vi "_JKISMQFGV.vi"(6 "Operation":T3, 8 "Error in":errorcluster caption="Error in (no error)", 9 "create if not found? (T)":bool=TRUE, 11 "Name(\"\" to use uuid) in":string) -> (0 "Error out":errorcluster, 1 "Boolean":bool, 2 "Name":string[](array[string]), 3 "Array":T1[](array[typedef]))   [LabVIEW 2014, in "JKI State Machine++.lvlib"]
uses:
  JKI State Machine++.lvlib
  _JKISMQFGVOPER.ctl
  _JKISMQ.ctl
  Typedef/_Cross JKISM State Data.ctl
  Typedef/_JKISM_MSG_TYPE.ctl
  Typedef/_Cross JKISM State Response.ctl
  Typedef/_JKISM_MODE.ctl
  Typedef/_JKISM Status Change Event Data.ctl
  FGV-BroadcastRegistry/Operation-BroadcastRegistry.ctl
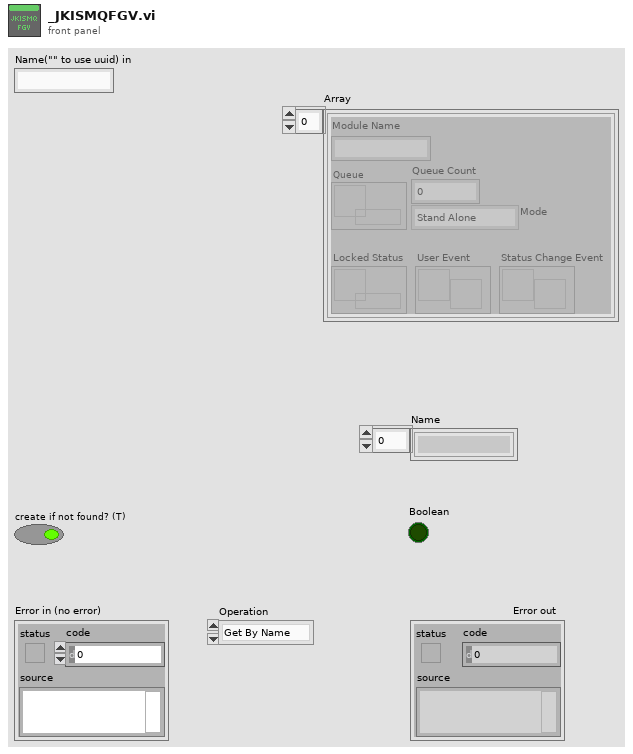
[diagram p1: front panel]
types:
  T1 = typedef "JKI State Machine++.lvlib/_JKISMQ.ctl" = cluster{"Module Name":string, "Queue":refnum<queue>, "Locked Status":refnum<data-value>, "Mode":T2, "User Event":refnum<user-event>, "Queue Count":i32, "Status Change Event":refnum<user-event>}
  T2 = typedef "JKI State Machine++.lvlib/_JKISM_MODE.ctl" = enum16{"Stand Alone", "JKISM", "Action Worker"}
  T3 = typedef "JKI State Machine++.lvlib/_JKISMQFGVOPER.ctl" = enum16{"Get By Name", "List", "Check If Name Exists", "Release", "Module Status", "Create Status Event Handler", "Destroy Status Event Handler"}
  T4 = typedef "JKI State Machine++.lvlib/Operation-BroadcastRegistry.ctl" = enum16{"Delete Source Module", "Delete Target Module", "Remove Module", "Register", "Unregister", "Check"}
  T5 = typedef "JKI State Machine++.lvlib/_JKISM Status Change Event Data.ctl" = cluster{"ModuleName":string, "Status":string, "Arguments":string}
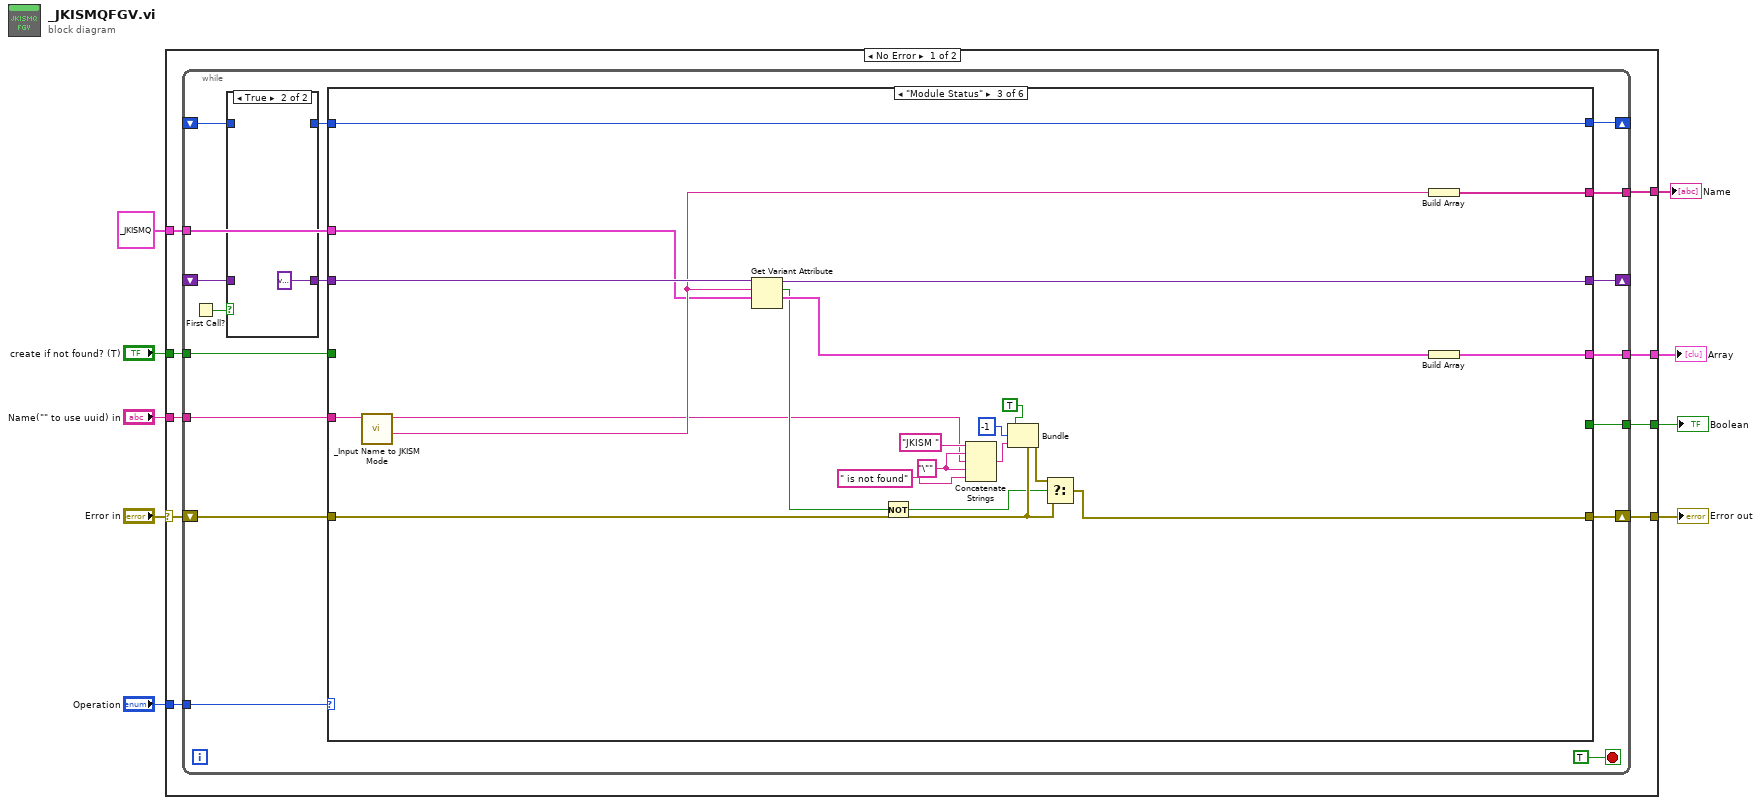
[diagram p0: block diagram]
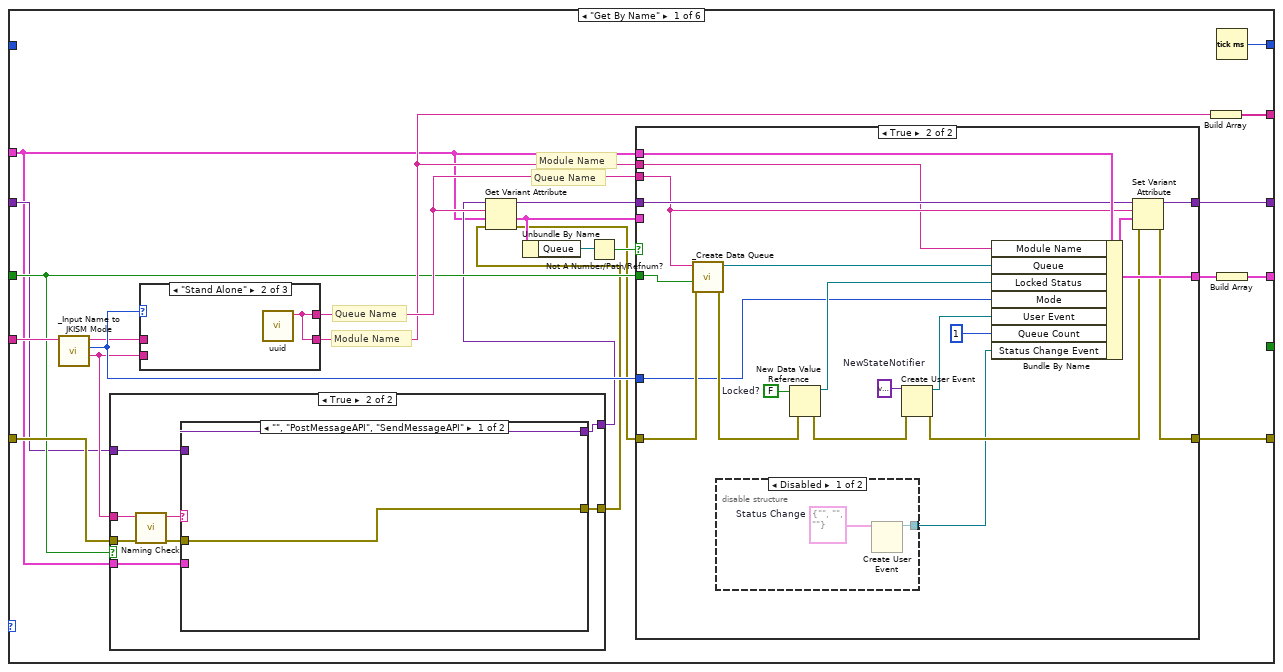
[diagram p3: hidden frame]
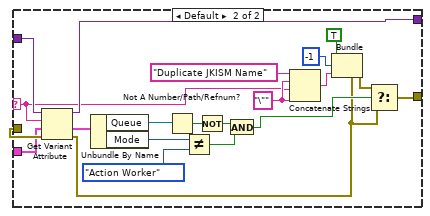
[diagram p5: hidden frame]
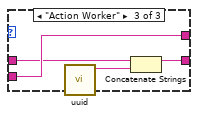
[diagram p7: hidden frame]
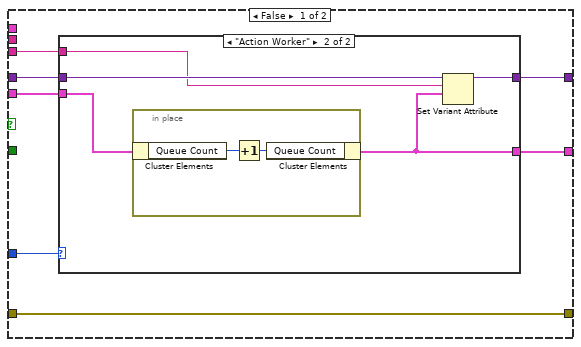
[diagram p8: hidden frame]
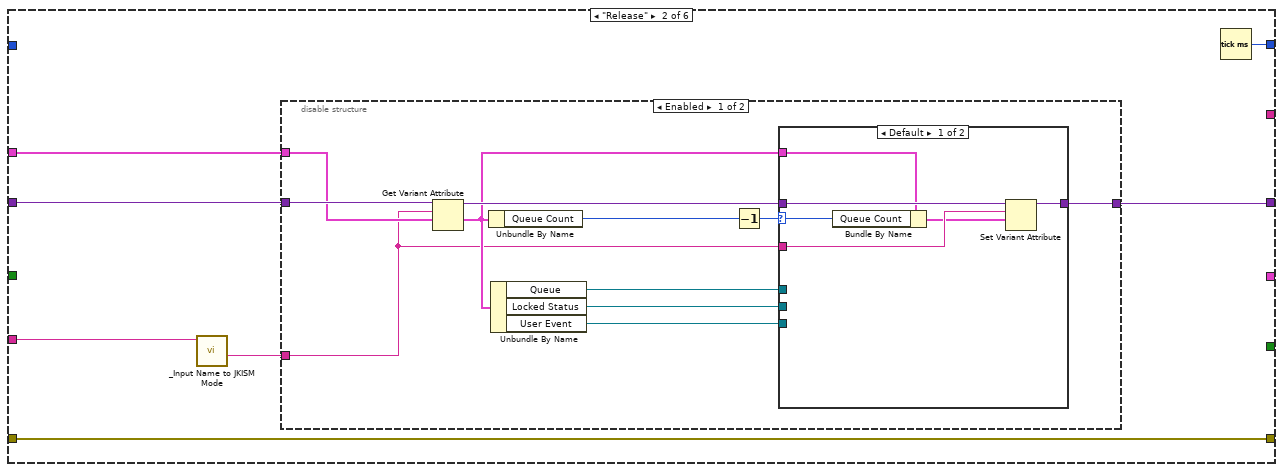
[diagram p11: hidden frame]
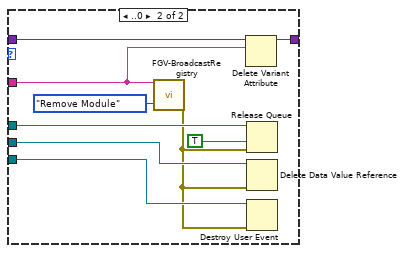
[diagram p12: hidden frame]
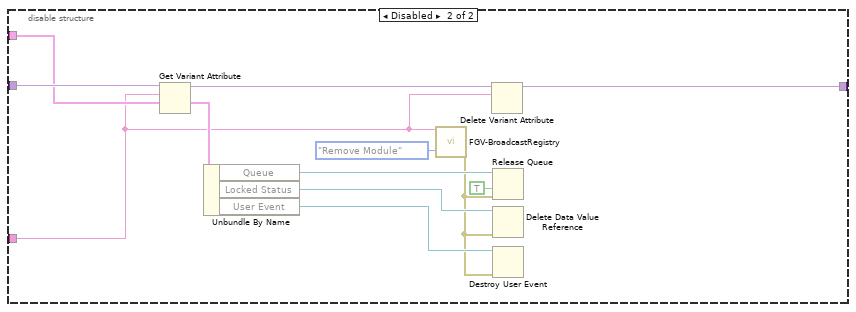
[diagram p13: hidden frame]
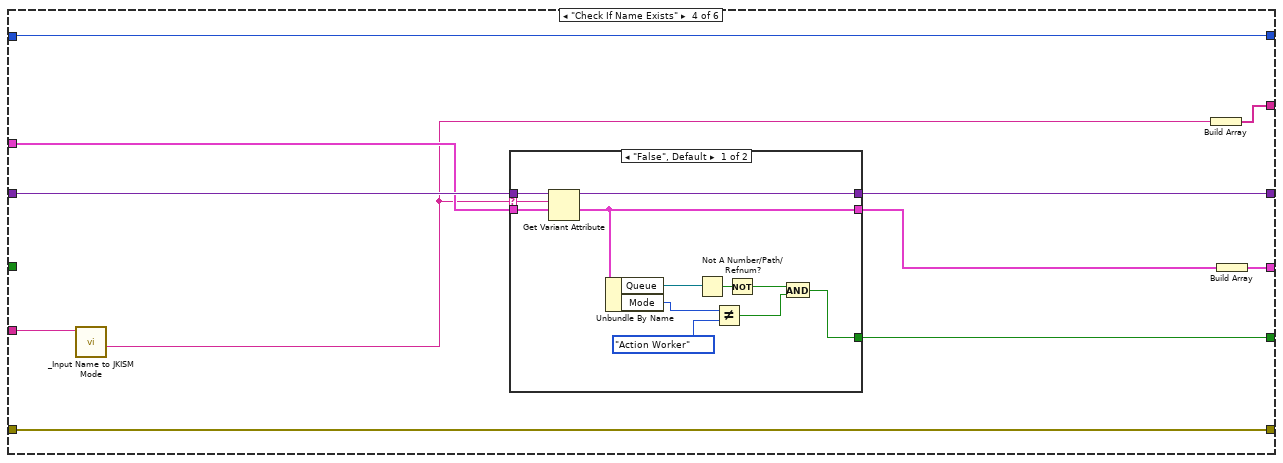
[diagram p14: hidden frame]
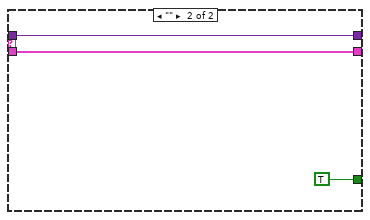
[diagram p15: hidden frame]
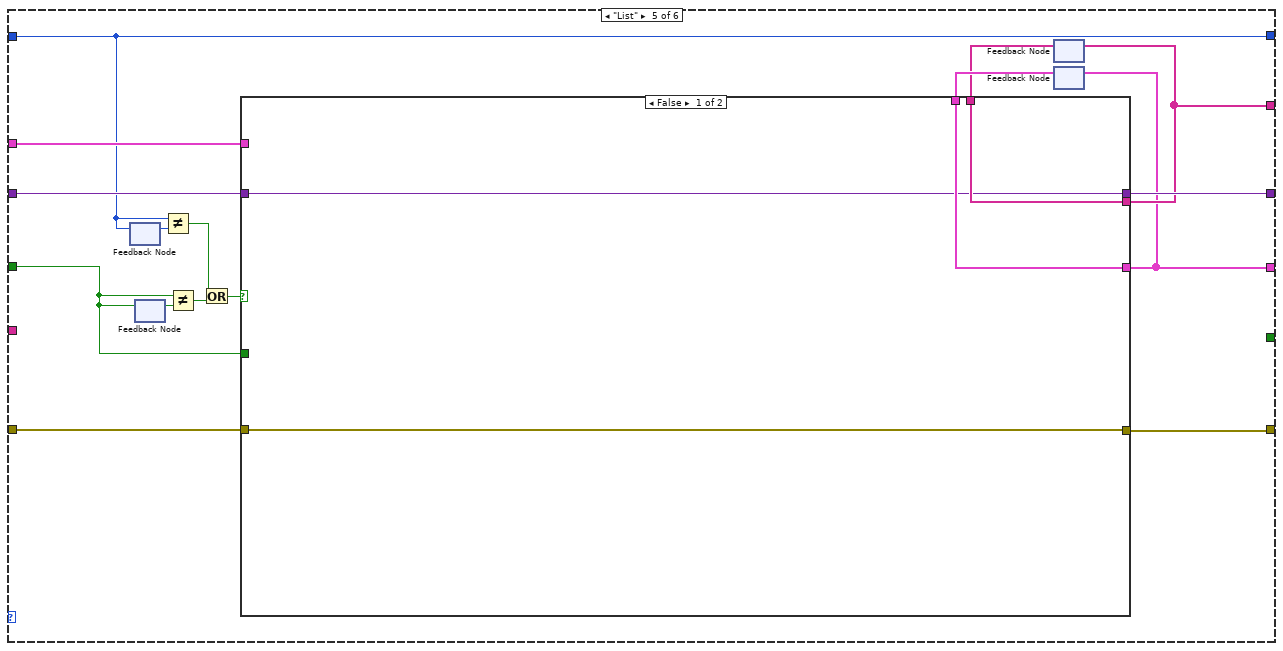
[diagram p16: hidden frame]
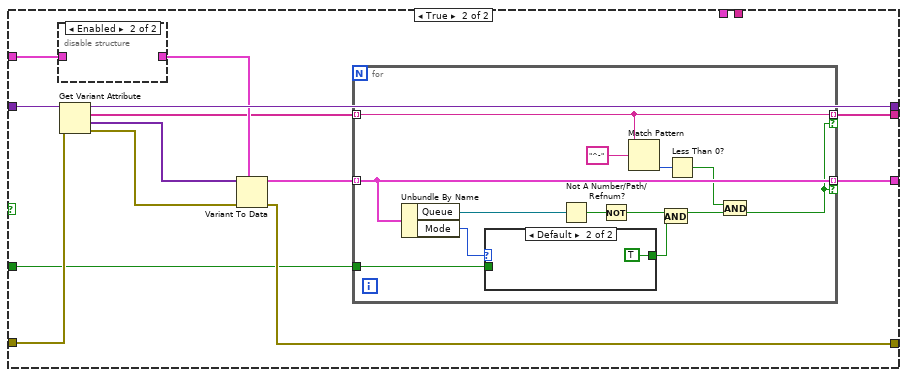
[diagram p17: hidden frame]
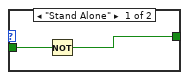
[diagram p18: hidden frame]
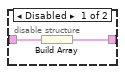
[diagram p19: hidden frame]
diagram:
  n1 = case shown="No Error" "Error in" {
    selector: "Error in" -> [w15 w285]
    tunnel: "Operation" -> [w18 _]
    tunnel: "Name(\"\" to use uuid) in" -> [w17 _]
    tunnel: "create if not found? (T)" -> [w16 _]
    tunnel: [w14 w285] -> w5
    tunnel: [w13 _] -> w4
    tunnel: T1 {"Module Name"="", "Queue"=refnum, "Locked Status"=refnum, "Mode"=enum."Stand Alone", "User Event"=refnum, "Queue Count"=0, "Status Change Event"=refnum} ("JKISMQ") -> [w12 _]
    tunnel: [w11 _] -> w2
    tunnel: [w10 _] -> w1
    frame No Error {
      n2 = while {
        tunnel: w18 -> [w34]
        tunnel: w17 -> [w33]
        tunnel: w16 -> [w32]
        tunnel: [w31] -> w11
        shift-right: [w27] -> _
        shift-left: _ -> [w29]
        shift-right: [w25] -> w14
        shift-left: w15 -> [w26]
        tunnel: [w24] -> w13
        tunnel: w12 -> [w23]
        tunnel: [w22] -> w10
        shift-right: [w21] -> _
        shift-left: _ -> [w19]
        stop <- TRUE stop-if-true
        n3 = First Call?() -> (First Call?: T/F=w30:bool)
        n4 = case shown="True" w30 {
          tunnel: [w37 variant] -> w28
          tunnel: w29 -> [w37 _]
          tunnel: [w36 _] -> w20
          tunnel: w19 -> [w36 _]
          frame False {
          }
          frame True {
          }
        }
        n5 = case shown="\"Module Status\"" w34 {
          tunnel: w33 -> [w52 w141 w203 w207 _ _]
          tunnel: w32 -> [w44 _ _ _ w238 _]
          tunnel: [w54 _ w200 w210 w233 _] -> w31
          tunnel: w28 -> [w43 w144 w204 w215 w246 w284]
          tunnel: [w59 w143 w202 w214 w245 w284] -> w27
          tunnel: w26 -> [w46 w145 w191 w212 w243 w283]
          tunnel: [w55 w145 w188 w212 w242 w283] -> w25
          tunnel: [w53 _ w198 w209 w234 _] -> w24
          tunnel: w23 -> [w41 w142 w196 w211 w244 _]
          tunnel: [_ _ _ w208 _ _] -> w22
          tunnel: w20 -> [_ _ w197 w205 w240 w282]
          tunnel: [w47 w139 w197 w205 w240 w282] -> w21
          frame "Get By Name" {
            # "Module Name"
            # "Queue Name"
            # "Module Name"
            # "Queue Name"
            n6 = call "_Input Name to JKISM Mode.vi"("String"=w52) -> ("Queue Name"=w45:string, "JKISM Mode"=w51:T2, "String(dup)"=w50:string)  [unwired: 8 in]
            n7 = case shown="True" w44 {
              tunnel: w45 -> [_ w65]
              tunnel: [w63 w71] -> w40
              tunnel: w46 -> [w63 w67]
              tunnel: w43 -> [w62 w70]
              tunnel: [w62 w69] -> w42
              tunnel: w41 -> [_ w68]
              frame False {
              }
              frame True {
                n8 = call "Naming Check.vi"("error in (no error)"=w67, "Name(\"\" to use uuid)"=w65) -> ("error out"=w66:errorcluster, "Name(dup)"=w64:string)  [unwired: 8 in]
                n9 = case shown="\"\", \"PostMessageAPI\", \"SendMessageAPI\"" w64 {
                  selector: w64 -> [_ w74]
                  tunnel: [w72 w94] -> w71
                  tunnel: w66 -> [w72 w77]
                  tunnel: w70 -> [w73 w79]
                  tunnel: [w73 w78] -> w69
                  tunnel: w68 -> [_ w75]
                  frame "", "PostMessageAPI", "SendMessageAPI" {
                  }
                  frame Default {
                    w88 = "\"" ("string")
                    n10 = Get Variant Attribute(Variant=w79, name=w74, default value (empty Variant)=w75, error in=w77) -> (duplicate Variant=w78:variant, value=w81:T1, error out=w76:errorcluster)  [unwired: 1 out]
                    n11 = Unbundle By Name(w81) -> ("Queue"=w82:refnum<queue>, "Mode"=w85:T2)
                    n12 = Not A Number/Path/Refnum?(number/path/refnum=w82) -> (NaN/Path/Refnum?=w83:bool)
                    n13 = Not Equal?(x=w85, y=_JKISM_MODE."Action Worker") -> (x != y?=w87:bool)
                    n14 = Not(x=w83) -> (.not. x?=w84:bool)
                    n15 = And(x=w84, y=w87) -> (x .and. y?=w80:bool)
                    n16 = Concatenate Strings("Duplicate JKISM Name" ("String to Prepend to source (\"\")"), w88, w74, w88) -> (w89:string)
                    n17 = Bundle(cluster=w76, "status"=TRUE, "code"=-1, "source"=w89) -> (w93:errorcluster)
                    n18 = Select(t=w93, s=w80, f=w76) -> (s? t:f=w94:errorcluster)
                  }
                }
              }
            }
            n19 = case shown="\"Stand Alone\"" w51 {
              tunnel: [w95 w96 w100] -> w49
              tunnel: [w95 w96 w97] -> w48
              tunnel: w50 -> [w95 _ w99]
              tunnel: w45 -> [_ _ w100]
              frame "JKISM" {
              }
              frame "Stand Alone" {
                n20 = call "uuid.vi"() -> ("UUID"=w96:string)  [unwired: 11 in]
              }
              frame "Action Worker" {
                n21 = call "uuid.vi"() -> ("UUID"=w98:string)  [unwired: 11 in]
                n22 = Concatenate Strings(w99, w98) -> (w97:string)
              }
            }
            n23 = Get Variant Attribute(Variant=w42, name=w49, default value (empty Variant)=w41, error in=w40) -> (duplicate Variant=w60:variant, value=w58:T1, error out=w39:errorcluster)  [unwired: 1 out]
            n24 = Unbundle By Name(w58) -> ("Queue"=w57:refnum<queue>)
            n25 = Not A Number/Path/Refnum?(number/path/refnum=w57) -> (NaN/Path/Refnum?=w56:bool)
            n26 = case shown="True" w56 {
              tunnel: w44 -> [_ w135]
              tunnel: [w103 w129] -> w61
              tunnel: w49 -> [w101 w119]
              tunnel: w41 -> [_ w132]
              tunnel: w60 -> [w104 w131]
              tunnel: [w105 w130] -> w59
              tunnel: w58 -> [w102 _]
              tunnel: w39 -> [w107 w128]
              tunnel: [w107 w126] -> w55
              tunnel: w51 -> [w106 w121]
              tunnel: w48 -> [_ w118]
              frame False {
                n27 = case shown="\"Action Worker\"" w106 {
                  tunnel: [w109 w113] -> w105
                  tunnel: w104 -> [w109 w114]
                  tunnel: [w108 w110] -> w103
                  tunnel: w102 -> [w108 w111]
                  tunnel: w101 -> [_ w112]
                  frame Default {
                  }
                  frame "Action Worker" {
                    n28 = in-place {
                      n29 = in-place-cluster #1(w111) -> ("Queue Count"=w116:i32)
                      n30 = Increment(x=w116) -> (x+1=w115:i32)
                      n31 = in-place-cluster #1("Queue Count"=w115) -> (w110:T1)
                    }
                    n32 = Set Variant Attribute(Variant=w114, name=w112, value=w110) -> (Variant out=w113:variant)  [unwired: 1 in, 2 out]
                  }
                }
              }
              frame True {
                w125 = variant  # NewStateNotifier
                w136 = FALSE  # Locked?
                n33 = call "_Create Data Queue.vi"("error in (no error)"=w128, "create if not found? (T)"=w135, "Name"=w119) -> ("error out"=w127:errorcluster, "Queue out"=w134:refnum<queue>)  [unwired: 6 in, 1 out]
                n34 = disable-structure shown="Disabled" {
                  disable-tunnel: [w137 _] -> w117
                  frame Disabled {
                    w138 = T5 {"ModuleName"="", "Status"="", "Arguments"=""}  # Status Change
                    n35 = Create User Event(user event datatype=w138) -> (user event=w137:refnum<user-event>)  [unwired: 1 in, 1 out]
                  }
                  frame Enabled {
                  }
                }
                n36 = New Data Value Reference(data value=w136, error in=w127) -> (data value reference=w133:refnum<data-value>, error out=w124:errorcluster)
                n37 = Create User Event(user event datatype=w125, error in=w124) -> (user event=w123:refnum<user-event>, error out=w122:errorcluster)
                n38 = Bundle By Name(cluster=w132, "Module Name"=w118, "Queue"=w134, "Locked Status"=w133, "Mode"=w121, "User Event"=w123, "Queue Count"=1, "Status Change Event"=w117) -> (w129:T1)
                n39 = Set Variant Attribute(Variant=w131, name=w119, value=w129, error in=w122) -> (Variant out=w130:variant, error out=w126:errorcluster)  [unwired: 1 out]
              }
            }
            n40 = Build Array(w48) -> (w53:string[])
            n41 = Tick Count (ms)() -> (millisecond timer value=w47:u32)
            n42 = Build Array(w61) -> (w54:T1[])
          }
          frame "Release" {
            n43 = call "_Input Name to JKISM Mode.vi"("String"=w141) -> ("Queue Name"=w140:string)  [unwired: 8 in, 2 out]
            n44 = disable-structure shown="Enabled" {
              disable-tunnel: w144 -> [w153 w180]
              disable-tunnel: [w149 w178] -> w143
              disable-tunnel: w142 -> [w148 w177]
              disable-tunnel: w140 -> [w146 w175]
              frame Enabled {
                n45 = Get Variant Attribute(Variant=w153, name=w146, default value (empty Variant)=w148) -> (duplicate Variant=w150:variant, value=w147:T1)  [unwired: 1 in, 2 out]
                n46 = Unbundle By Name(w147) -> ("Queue Count"=w152:i32)
                n47 = Unbundle By Name(w147) -> ("Queue"=w156:refnum<queue>, "Locked Status"=w155:refnum<data-value>, "User Event"=w154:refnum<user-event>)
                n48 = Decrement(x=w152) -> (x-1=w151:i32)
                n49 = case shown="Default" w151 {
                  selector: w151 -> [w157 _]
                  tunnel: w156 -> [_ w171]
                  tunnel: w155 -> [_ w169]
                  tunnel: w154 -> [_ w168]
                  tunnel: w146 -> [w159 w163]
                  tunnel: w150 -> [w162 w165]
                  tunnel: [w161 w164] -> w149
                  tunnel: w147 -> [w160 _]
                  frame Default {
                    n50 = Bundle By Name(cluster=w160, "Queue Count"=w157) -> (w158:T1)
                    n51 = Set Variant Attribute(Variant=w162, name=w159, value=w158) -> (Variant out=w161:variant)  [unwired: 1 in, 2 out]
                  }
                  frame ..0 {
                    n52 = call "FGV-BroadcastRegistry.vi"("Source"=w163, "Operation"=Operation-BroadcastRegistry."Remove Module") -> ("Error out"=w166:errorcluster)  [unwired: 11 in, 2 out]
                    n53 = Delete Variant Attribute(6:w163, 7:w165) -> (3:w164:variant)  [unwired: 1 in, 2 out]
                    n54 = Release Queue(queue=w171, force destroy? (F)=TRUE, error in (no error)=w166) -> ()  [unwired: 3 out]
                    n55 = Delete Data Value Reference(data value reference=w169, error in=w166) -> ()  [unwired: 2 out]
                    n56 = Destroy User Event(user event=w168, error in=w166) -> ()  [unwired: 1 out]
                  }
                }
              }
              frame Disabled {
                n57 = Get Variant Attribute(Variant=w180, name=w175, default value (empty Variant)=w177) -> (duplicate Variant=w179:variant, value=w176:T1)  [unwired: 1 in, 2 out]
                n58 = Unbundle By Name(w176) -> ("Queue"=w183:refnum<queue>, "Locked Status"=w182:refnum<data-value>, "User Event"=w181:refnum<user-event>)
                n59 = call "FGV-BroadcastRegistry.vi"("Source"=w175, "Operation"=Operation-BroadcastRegistry."Remove Module") -> ("Error out"=w172:errorcluster)  [unwired: 11 in, 2 out]
                n60 = Delete Variant Attribute(6:w175, 7:w179) -> (3:w178:variant)  [unwired: 1 in, 2 out]
                n61 = Release Queue(queue=w183, force destroy? (F)=TRUE, error in (no error)=w172) -> ()  [unwired: 3 out]
                n62 = Delete Data Value Reference(data value reference=w182, error in=w172) -> ()  [unwired: 2 out]
                n63 = Destroy User Event(user event=w181, error in=w172) -> ()  [unwired: 1 out]
              }
            }
            n64 = Tick Count (ms)() -> (millisecond timer value=w139:u32)
          }
          frame "Module Status" {
            w192 = "\"" ("string")
            n65 = call "_Input Name to JKISM Mode.vi"("String"=w203) -> ("Queue Name"=w199:string, "String(dup)"=w186:string)  [unwired: 8 in, 1 out]
            n66 = Get Variant Attribute(Variant=w204, name=w199, default value (empty Variant)=w196) -> (duplicate Variant=w202:variant, found=w190:bool, value=w201:T1)  [unwired: 1 in, 1 out]
            n67 = Not(x=w190) -> (.not. x?=w189:bool)
            n68 = Concatenate Strings("JKISM " ("String to Prepend to source (\"\")"), w192, w186, w192, " is not found" ("string")) -> (w193:string)
            n69 = Bundle(cluster=w191, "status"=TRUE, "code"=-1, "source"=w193) -> (w195:errorcluster)
            n70 = Select(t=w195, s=w189, f=w191) -> (s? t:f=w188:errorcluster)
            n71 = Build Array(w199) -> (w198:string[])
            n72 = Build Array(w201) -> (w200:T1[])
          }
          frame "Check If Name Exists" {
            n73 = call "_Input Name to JKISM Mode.vi"("String"=w207) -> ("Queue Name"=w206:string)  [unwired: 8 in, 2 out]
            n74 = case shown="\"False\", Default" w206 {
              selector: w206 -> [w224 _]
              tunnel: w215 -> [w227 w230]
              tunnel: [w226 w230] -> w214
              tunnel: [w223 w228] -> w213
              tunnel: w211 -> [w225 w228]
              tunnel: [w219 TRUE] -> w208
              frame "False", Default {
                n75 = Get Variant Attribute(Variant=w227, name=w224, default value (empty Variant)=w225) -> (duplicate Variant=w226:variant, value=w223:T1)  [unwired: 1 in, 2 out]
                n76 = Unbundle By Name(w223) -> ("Queue"=w222:refnum<queue>, "Mode"=w218:T2)
                n77 = Not A Number/Path/Refnum?(number/path/refnum=w222) -> (NaN/Path/Refnum?=w221:bool)
                n78 = Not Equal?(x=w218, y=_JKISM_MODE."Action Worker") -> (x != y?=w216:bool)
                n79 = Not(x=w221) -> (.not. x?=w220:bool)
                n80 = And(x=w220, y=w216) -> (x .and. y?=w219:bool)
              }
              frame "" {
              }
            }
            n81 = Build Array(w206) -> (w209:string[])
            n82 = Build Array(w213) -> (w210:T1[])
          }
          frame "List" {
            n83 = feedback-in #2(w240) -> ()
            n84 = feedback #2() -> (w241:u32)  [unwired: 1 in]
            n85 = feedback #3() -> (w239:bool)  [unwired: 1 in]
            n86 = feedback-in #3(w238) -> ()
            n87 = Not Equal?(x=w240, y=w241) -> (x != y?=w236:bool)
            n88 = Not Equal?(x=w238, y=w239) -> (x != y?=w237:bool)
            n89 = Or(x=w236, y=w237) -> (x .or. y?=w235:bool)
            n90 = feedback #4() -> (w231:string[])  [unwired: 1 in]
            n91 = feedback #5() -> (w232:T1[])  [unwired: 1 in]
            n92 = case shown="False" w235 {
              tunnel: w246 -> [w248 w263]
              tunnel: [w248 w262] -> w245
              tunnel: w244 -> [_ w260]
              tunnel: [w249 w256] -> w234
              tunnel: [w250 w255] -> w233
              tunnel: w243 -> [w247 w253]
              tunnel: [w247 w252] -> w242
              tunnel: w238 -> [_ w251]
              tunnel: w232 -> [w250 _]
              tunnel: w231 -> [w249 _]
              frame False {
              }
              frame True {
                n93 = disable-structure shown="Enabled" {
                  disable-tunnel: w260 -> [w281 _]
                  disable-tunnel: [w280 _] -> w259
                  frame Disabled {
                    n94 = Build Array(w281) -> (w280:T1[])
                  }
                  frame Enabled {
                  }
                }
                n95 = Get Variant Attribute(Variant=w263, error in=w253) -> (duplicate Variant=w262:variant, names=w257:string[], values=w261:variant[], error out=w254:errorcluster)  [unwired: 2 in]
                n96 = Variant To Data(error in=w254, type=w259, Variant=w261) -> (data=w258:T1[], error out=w252:errorcluster)
                n97 = for {
                  tunnel: w258 -> [w276] mode=indexing
                  tunnel: w257 -> [w267] mode=indexing
                  tunnel: [w267] -> w256 mode=indexing if=w268
                  tunnel: [w276] -> w255 mode=indexing if=w268
                  tunnel: w251 -> [w269]
                  n98 = Unbundle By Name(w276) -> ("Queue"=w275:refnum<queue>, "Mode"=w271:T2)
                  n99 = case shown="Default" w271 {
                    tunnel: [w277 TRUE] -> w270
                    tunnel: w269 -> [w278 _]
                    frame "Stand Alone" {
                      n100 = Not(x=w278) -> (.not. x?=w277:bool)
                    }
                    frame Default {
                    }
                  }
                  n101 = Not A Number/Path/Refnum?(number/path/refnum=w275) -> (NaN/Path/Refnum?=w274:bool)
                  n102 = Not(x=w274) -> (.not. x?=w272:bool)
                  n103 = Match Pattern(string=w267, regular expression="^-") -> (offset past match=w265:i32)  [unwired: 1 in, 3 out]
                  n104 = And(x=w272, y=w270) -> (x .and. y?=w273:bool)
                  n105 = Less Than 0?(x=w265) -> (x < 0?=w264:bool)
                  n106 = And(x=w264, y=w273) -> (x .and. y?=w268:bool)
                }
              }
            }
            n107 = feedback-in #4(w234) -> ()
            n108 = feedback-in #5(w233) -> ()
          }
          frame Default {
          }
        }
      }
    }
    frame Error {
    }
  }
  "Error out" <- w5
  "Name" <- w4
  "Array" <- w2
  "Boolean" <- w1
